vi "LEITURA VALORES SERVER.vi"() -> ()   [LabVIEW 2019]
panel:
  in  "stop":bool
  in  "tam":dbl
  out "VALORES":string[](array[string])
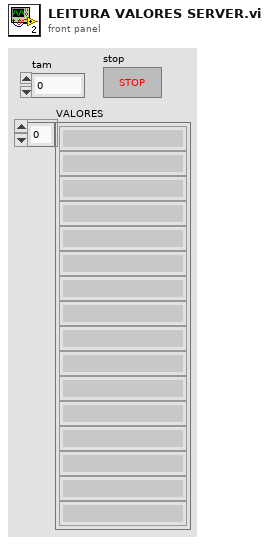
[diagram p1: front panel]
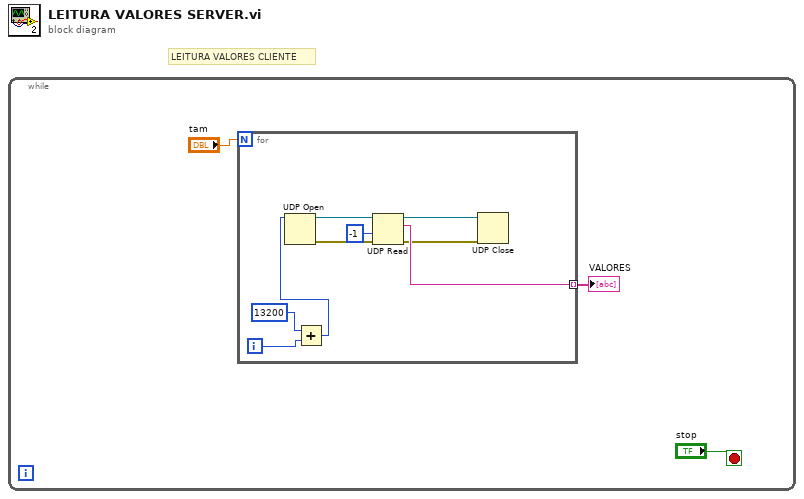
[diagram p0: block diagram]
diagram:
  # "LEITURA VALORES CLIENTE"
  n1 = while {
    stop <- "stop" stop-if-true
    n2 = for {
      N: "tam" -> [_]
      tunnel: [w5] -> w2 mode=indexing
      i -> [w11]
      n3 = Add(x=u16 13200 ("port"), y=w11) -> (x+y=w10:i32)
      n4 = UDP Open(11:w10) -> (port=w9:refnum<k16>, 0:w7:errorcluster)  [unwired: 4 in, 1 out]
      n5 = UDP Read(connection ID=w9, timeout ms (25000)=-1, 8:w7) -> (data out=w5:string, error out=w4:errorcluster, 3:w8:refnum<k16>)  [unwired: 1 in, 2 out]
      n6 = UDP Close(connection ID=w8, 8:w4) -> ()  [unwired: 2 out]
    }
    "VALORES" <- w2
  }
